vi "CTL_Set_Resistor ValueRev3.vi"(10 "Level IN inches":dbl, 11 "Spec Range":T1) -> (3 "Resistor":dbl)   [LabVIEW 2024]
uses:
  Control Definitions/Def Spec RNG.ctl
  Control Definitions/Ded LUT_Status.ctl
panel:
  out "x .xor. y?":bool
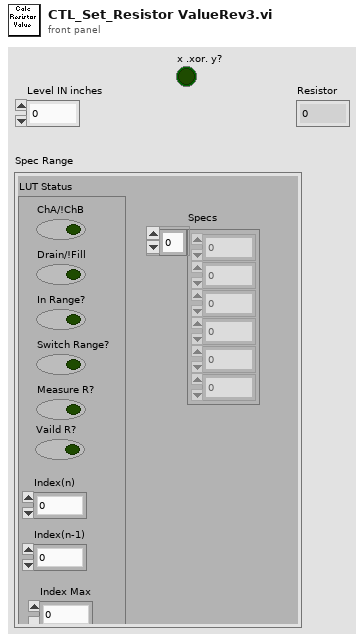
[diagram p1: front panel]
types:
  T1 = typedef "Def Spec RNG.ctl" = cluster{"Specs":dbl[], "LUT Status":T2}
  T2 = typedef "Ded LUT_Status.ctl" = cluster{"ChA/!ChB":bool, "Drain/!Fill":bool, "In Range?":bool, "Switch Range?":bool, "Measure R?":bool, "Vaild R?":bool, "Index(n)":i32, "Index(n-1)":i32, "Index Max":i32}
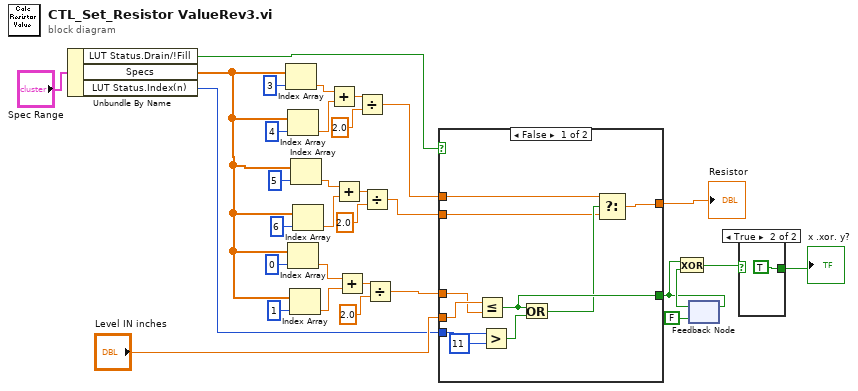
[diagram p0: block diagram]
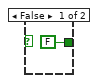
[diagram p2: hidden frame]
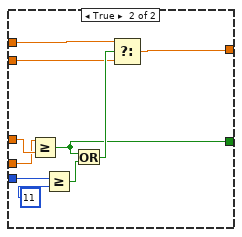
[diagram p3: hidden frame]
diagram:
  n1 = Unbundle By Name("Spec Range") -> ("LUT Status.Drain/!Fill"=w14:bool, "Specs"=w2:dbl[], "LUT Status.Index(n)"=w15:i32)
  n2 = Index Array(array=w2, index=3) -> (element=w29:dbl)
  n3 = Index Array(array=w2, index=4) -> (element=w30:dbl)
  n4 = Index Array(array=w2, index=0) -> (element=w21:dbl)
  n5 = Index Array(array=w2, index=1) -> (element=w20:dbl)
  n6 = Index Array(array=w2, index=5) -> (element=w5:dbl)
  n7 = Index Array(array=w2, index=6) -> (element=w6:dbl)
  n8 = Add(x=w29, y=w30) -> (x+y=w31:dbl)
  n9 = Add(x=w5, y=w6) -> (x+y=w7:dbl)
  n10 = Add(x=w21, y=w20) -> (x+y=w22:dbl)
  n11 = Divide(x=w31, y=2.0) -> (x/y=w16:dbl)
  n12 = Divide(x=w7, y=2.0) -> (x/y=w1:dbl)
  n13 = Divide(x=w22, y=2.0) -> (x/y=w18:dbl)
  n14 = case shown="False" w14 {
    tunnel: [w40 w52] -> w19
    tunnel: w18 -> [w41 w46]
    tunnel: "Level IN inches" -> [w42 w45]
    tunnel: w16 -> [w39 w44]
    tunnel: w15 -> [w37 w49]
    tunnel: [w38 w47] -> w11
    tunnel: w1 -> [w33 w43]
    frame False {
      n15 = Less Or Equal?(x=w42, y=w41) -> (x <= y?=w38:bool)
      n16 = Greater?(x=w37, y=11) -> (0:w34:bool)
      n17 = Or(x=w38, y=w34) -> (x .or. y?=w35:bool)
      n18 = Select(t=w39, s=w35, f=w33) -> (s? t:f=w40:dbl)
    }
    frame True {
      n19 = Greater Or Equal?(x=w45, y=w46) -> (x >= y?=w47:bool)
      n20 = Greater Or Equal?(x=w49, y=11) -> (x >= y?=w50:bool)
      n21 = Or(x=w47, y=w50) -> (x .or. y?=w51:bool)
      n22 = Select(t=w44, s=w51, f=w43) -> (s? t:f=w52:dbl)
    }
  }
  "Resistor" <- w19
  n23 = feedback-in #1(w11) -> ()
  n24 = feedback #1(FALSE) -> (w12:bool)
  n25 = Exclusive Or(1:w12, 2:w11) -> (0:w10:bool)
  n26 = case shown="True" w10 {
    tunnel: [FALSE ("x .xor. y?") TRUE ("x .xor. y?")] -> w9
    frame False {
    }
    frame True {
    }
  }
  "x .xor. y?" <- w9
